vi "Categorize Timestamp Relativity.vi"(1 "Today's Time Stamp":timestamp, 2 "Second Time Stamp":timestamp) -> (0 "First Relative to Today's Time Stamp":string)   [LabVIEW 2011]
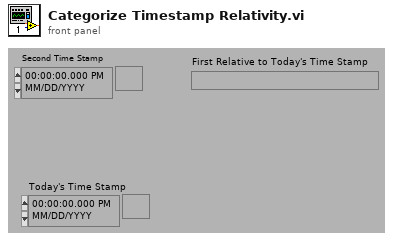
[diagram p1: front panel]
types:
  T1 = cluster{"second":i32, "minute":i32, "hour":i32, "day of month":i32, "month":i32, "year":i32, "day of week":i32, "day of year":i32, "is DST":i32}
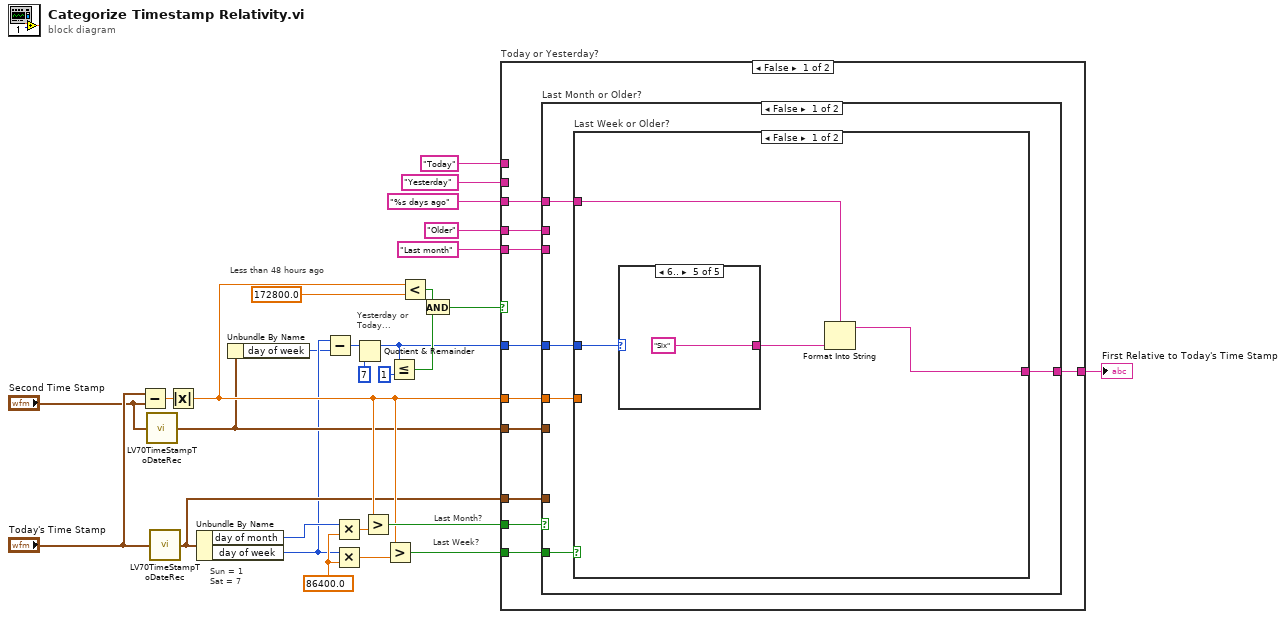
[diagram p0: block diagram]
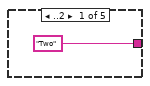
[diagram p2: hidden frame]
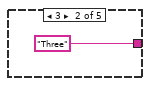
[diagram p3: hidden frame]
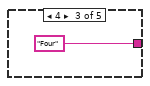
[diagram p4: hidden frame]
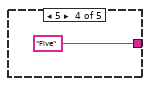
[diagram p5: hidden frame]
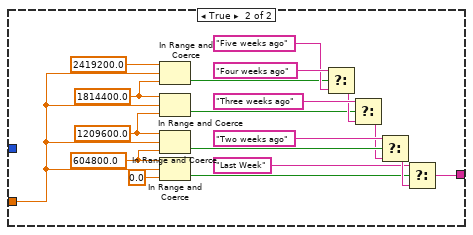
[diagram p6: hidden frame]
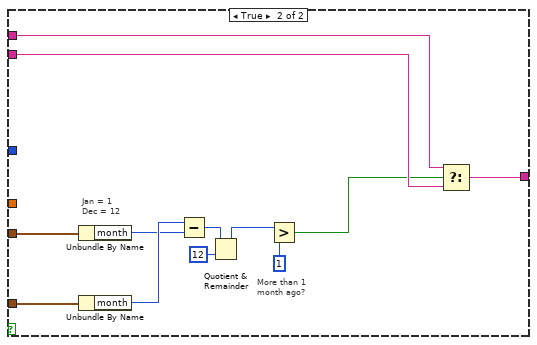
[diagram p7: hidden frame]
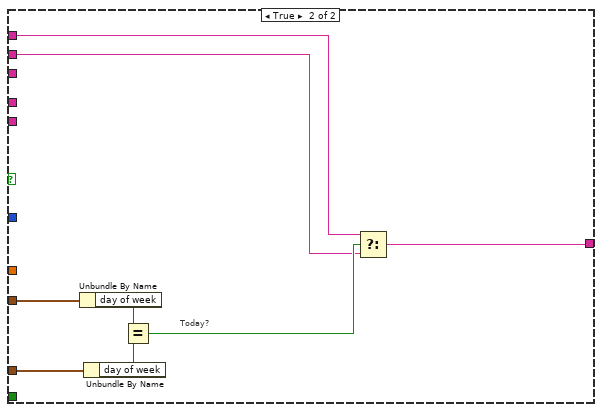
[diagram p8: hidden frame]
diagram:
  w9 = 86400.0 ("upper limit")
  # "Yesterday or\nToday..."
  # "Less than 48 hours ago"
  # "Last Week?"
  # "Last Month?"
  # "Sun = 1\nSat = 7"
  n1 = Subtract(x="Today's Time Stamp", y="Second Time Stamp") -> (x-y=w23:dbl)
  n2 = call <vilib>:"LV70TimeStampToDateRec.vi"("time stamp"="Second Time Stamp") -> ("date time rec"=w11:T1)
  n3 = call <vilib>:"LV70TimeStampToDateRec.vi"("time stamp"="Today's Time Stamp") -> ("date time rec"=w12:T1)
  n4 = Absolute Value(x=w23) -> (abs(x)=w15:dbl)
  n5 = Unbundle By Name(w12) -> ("day of month"=w10:i32, "day of week"=w7:i32)
  n6 = Unbundle By Name(w11) -> ("day of week"=w4:i32)
  n7 = Subtract(x=w7, y=w4) -> (x-y=w3:i32)
  n8 = Multiply(x=w10, y=w9) -> (x*y=w27:dbl)
  n9 = Multiply(x=w7, y=w9) -> (x*y=w25:dbl)
  n10 = Quotient & Remainder(x=w3, y=7) -> (x-y*floor(x/y)=w2:i32)  [unwired: 1 out]
  n11 = Greater?(x=w15, y=w27) -> (0:w26:bool)
  n12 = Greater?(x=w15, y=w25) -> (0:w24:bool)
  n13 = Less Or Equal?(x=w2, y=1) -> (x <= y?=w5:bool)
  n14 = Less?(x=w15, y=172800.0 ("upper limit")) -> (x < y?=w14:bool)
  n15 = And(x=w14, y=w5) -> (x .and. y?=w17:bool)
  n16 = case "Today or Yesterday?" shown="False" w17 {
    tunnel: [w37 w91] -> w28
    tunnel: w26 -> [w38 _]
    tunnel: w24 -> [w34 _]
    tunnel: w11 -> [w36 w85]
    tunnel: w12 -> [w35 w86]
    tunnel: w15 -> [w33 _]
    tunnel: "Today" -> [_ w88]
    tunnel: "Yesterday" -> [_ w87]
    tunnel: "Older" -> [w32 _]
    tunnel: "Last month" -> [w31 _]
    tunnel: w2 -> [w30 _]
    tunnel: "%s days ago" -> [w29 _]
    frame False {
      n17 = case "Last Month or Older?" shown="False" w38 {
        tunnel: [w42 w83] -> w37
        tunnel: w36 -> [_ w76]
        tunnel: w35 -> [_ w77]
        tunnel: w34 -> [w43 _]
        tunnel: w33 -> [w41 _]
        tunnel: w32 -> [_ w79]
        tunnel: w31 -> [_ w78]
        tunnel: w30 -> [w40 _]
        tunnel: w29 -> [w39 _]
        frame False {
          n18 = case "Last Week or Older?" shown="False" w43 {
            tunnel: [w44 w68] -> w42
            tunnel: w41 -> [_ w54]
            tunnel: w40 -> [w47 _]
            tunnel: w39 -> [w46 _]
            frame False {
              n19 = case shown="6.." w47 {
                tunnel: ["Two" "Three" "Four" "Five" "Six"] -> w45
                frame ..2 {
                }
                frame 3 {
                }
                frame 4 {
                }
                frame 5 {
                }
                frame 6.. {
                }
              }
              n20 = Format Into String(format string=w46, w45) -> (resulting string=w44:string)  [unwired: 2 in, 1 out]
            }
            frame True {
              w53 = 1814400.0 ("upper limit")
              w57 = 1209600.0 ("upper limit")
              w67 = 604800.0 ("upper limit")
              n21 = In Range and Coerce(upper limit=2419200.0, x=w54, lower limit=w53) -> (In Range?=w55:bool)  [unwired: 1 out]
              n22 = In Range and Coerce(upper limit=w53, x=w54, lower limit=w57) -> (In Range?=w58:bool)  [unwired: 1 out]
              n23 = In Range and Coerce(upper limit=w57, x=w54, lower limit=w67) -> (In Range?=w64:bool)  [unwired: 1 out]
              n24 = In Range and Coerce(upper limit=w67, x=w54, lower limit=0.0) -> (In Range?=w65:bool)  [unwired: 1 out]
              n25 = Select(t="Four weeks ago", s=w55, f="Five weeks ago") -> (s? t:f=w61:string)
              n26 = Select(t="Three weeks ago", s=w58, f=w61) -> (s? t:f=w63:string)
              n27 = Select(t="Two weeks ago", s=w64, f=w63) -> (s? t:f=w71:string)
              n28 = Select(t="Last Week", s=w65, f=w71) -> (s? t:f=w68:string)
            }
          }
        }
        frame True {
          # "Jan = 1\nDec = 12"
          # "More than 1\nmonth ago?"
          n29 = Unbundle By Name(w76) -> ("month"=w75:i32)
          n30 = Unbundle By Name(w77) -> ("month"=w81:i32)
          n31 = Subtract(x=w81, y=w75) -> (x-y=w74:i32)
          n32 = Quotient & Remainder(x=w74, y=12) -> (x-y*floor(x/y)=w73:i32)  [unwired: 1 out]
          n33 = Greater?(x=w73, y=1) -> (0:w72:bool)
          n34 = Select(t=w79, s=w72, f=w78) -> (s? t:f=w83:string)
        }
      }
    }
    frame True {
      # "Today?"
      n35 = Unbundle By Name(w85) -> ("day of week"=w84:i32)
      n36 = Unbundle By Name(w86) -> ("day of week"=w90:i32)
      n37 = Equal?(x=w84, y=w90) -> (x = y?=w89:bool)
      n38 = Select(t=w88, s=w89, f=w87) -> (s? t:f=w91:string)
    }
  }
  "First Relative to Today's Time Stamp" <- w28
